vi "Set Default S Parameter Report Parameters.vi"() -> (2 "Report Variables":T1={"REPORT_TDR_PATH"="Sxx Report.TDR", "ROOT_PATH"="", "PLOT1_TDM_PATH"="", "REPORT_PDF_PATH"="", "PLOT1_RUN_ID"=1, "PLOT_STYLE"=0, "COMPANY_ID_TXT"="Summitek", "DATETIME_TXT"="", "OPERATOR_TXT"="", "SERIALNUMBER_TXT"="", "MODELNUMBER_TXT"="", "SEQID_TXT"="", "INSTRID_TXT"="", "CUSTOMTXT 1"="", "CUSTOMTXT 2"="", "CUSTOMTXT 3"="", "CUSTOMTXT 4"="", "CUSTOMTXT 5"="", "CUSTOMTXT 6"="", "CUSTOMTXT 7"="", "CUSTOMTXT 8"="", "CUSTOMTXT 9"="", "CUSTOMTXT 10"="", "PLOT1_LABEL_TXT"="", "PLOT1_Y_TXT"="", "PLOT1_X_TXT"="", "PLOT2_LABEL_TXT"="", "PLOT2_Y_TXT"="", "PLOT2_X_TXT"="", "REPORTFOOTER"="", "PLOT1_FORMAT"=0, "PLOT1_LINETYPE"=1, "PLOT1_CURVES"=[], "PLOT1_AUTO_X"=1, "PLOT1_XMIN"=0.0, "PLOT1_XMAX"=0.0, "PLOT1_X_UNIT"=2, "PLOT1_AUTO_Y"=1, "PLOT1_YMIN"=0.0, "PLOT1_YMAX"=0.0, "PLOT2_FORMAT"=0, "PLOT2_LINETYPE"=1, "PLOT2_CURVES"=[], "PLOT2_AUTO_X"=1, "PLOT2_XMIN"=0.0, "PLOT2_XMAX"=0.0, "PLOT2_X_UNIT"=2, "PLOT2_AUTO_Y"=1, "PLOT2_YMIN"=0.0, "PLOT2_YMAX"=0.0, "PRINTER"="", "CUSTOMTXT 11"="", "CUSTOMTXT 12"="", "CUSTOMTXT 13"="", "CUSTOMTXT 14"="", "CUSTOMTXT 15"="", "CUSTOMTXT 16"="", "CUSTOMTXT 17"="", "CUSTOMTXT 18"="", "CUSTOMTXT 19"="", "CUSTOMTXT 20"="", "Custom_Count"=0, "PLOT1_MARKERS"=[], "PLOT2_MARKERS"=[], "S2P"=1, "ASCII"=1} {"PLOT2_X_UNIT" items=["Hz", "kHz", "MHz", "GHz"]; "PLOT2_FORMAT" items=["Log Magnitude", "Phase", "Delay", "Linear Magnitude", "VSWR", "Insertion Loss", "Isolation", "Return Loss", "Expanded Phase"]; "PLOT1_X_UNIT" items=["Hz", "kHz", "MHz", "GHz"]; "PLOT1_FORMAT" items=["Log Magnitude", "Phase", "Delay", "Linear Magnitude", "VSWR", "Insertion Loss", "Isolation", "Return Loss", "Expanded Phase"]; "PLOT_STYLE" items=["PDF", "HTML"]})   [LabVIEW 2011]
uses:
  server/DIAdem/Datasheet/Datasheet Sxx Parameters.ctl
  server/DIAdem/Datasheet/Datasheet Sxx Plot Formats.ctl
  server/DIAdem/Datasheet/Datasheet Sxx Plot Control.ctl
  server/DIAdem/Datasheet/Datasheet Sxx Frequency Units.ctl
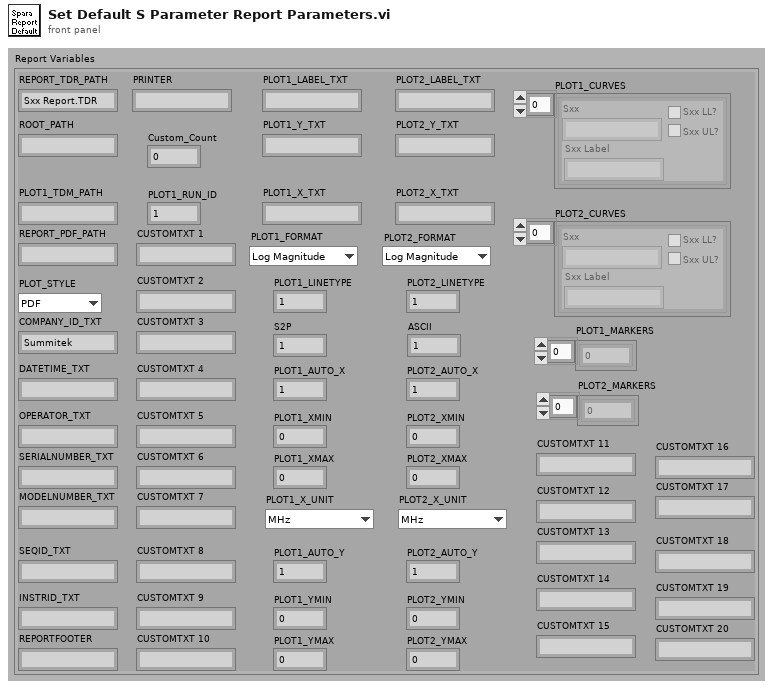
[diagram p1: front panel]
types:
  T1 = typedef "DATASHEET Sxx Parameters.ctl" = cluster{"REPORT_TDR_PATH":string, "ROOT_PATH":string, "PLOT1_TDM_PATH":string, "REPORT_PDF_PATH":string, "PLOT1_RUN_ID":i32, "PLOT_STYLE":u16, "COMPANY_ID_TXT":string, "DATETIME_TXT":string, "OPERATOR_TXT":string, "SERIALNUMBER_TXT":string, "MODELNUMBER_TXT":string, "SEQID_TXT":string, "INSTRID_TXT":string, "CUSTOMTXT 1":string, "CUSTOMTXT 2":string, "CUSTOMTXT 3":string, "CUSTOMTXT 4":string, "CUSTOMTXT 5":string, "CUSTOMTXT 6":string, "CUSTOMTXT 7":string, "CUSTOMTXT 8":string, "CUSTOMTXT 9":string, "CUSTOMTXT 10":string, "PLOT1_LABEL_TXT":string, "PLOT1_Y_TXT":string, "PLOT1_X_TXT":string, "PLOT2_LABEL_TXT":string, "PLOT2_Y_TXT":string, "PLOT2_X_TXT":string, "REPORTFOOTER":string, "PLOT1_FORMAT":T2, "PLOT1_LINETYPE":i32, "PLOT1_CURVES":T3[], "PLOT1_AUTO_X":i32, "PLOT1_XMIN":dbl, "PLOT1_XMAX":dbl, "PLOT1_X_UNIT":T4, "PLOT1_AUTO_Y":i32, "PLOT1_YMIN":dbl, "PLOT1_YMAX":dbl, "PLOT2_FORMAT":T2, "PLOT2_LINETYPE":i32, "PLOT2_CURVES":T3[], "PLOT2_AUTO_X":i32, "PLOT2_XMIN":dbl, "PLOT2_XMAX":dbl, "PLOT2_X_UNIT":T4, "PLOT2_AUTO_Y":i32, "PLOT2_YMIN":dbl, "PLOT2_YMAX":dbl, "PRINTER":string, "CUSTOMTXT 11":string, "CUSTOMTXT 12":string, "CUSTOMTXT 13":string, "CUSTOMTXT 14":string, "CUSTOMTXT 15":string, "CUSTOMTXT 16":string, "CUSTOMTXT 17":string, "CUSTOMTXT 18":string, "CUSTOMTXT 19":string, "CUSTOMTXT 20":string, "Custom_Count":i32, "PLOT1_MARKERS":dbl[], "PLOT2_MARKERS":dbl[], "S2P":i32, "ASCII":i32}
  T2 = typedef "DATASHEET Sxx Plot Formats.ctl" = u16
  T3 = typedef "DATASHEET Sxx Plot Control.ctl" = cluster{"Sxx":string, "Sxx LL?":bool, "Sxx UL?":bool, "Sxx Label":string}
  T4 = typedef "DATASHEET Sxx Frequency Units.ctl" = u16
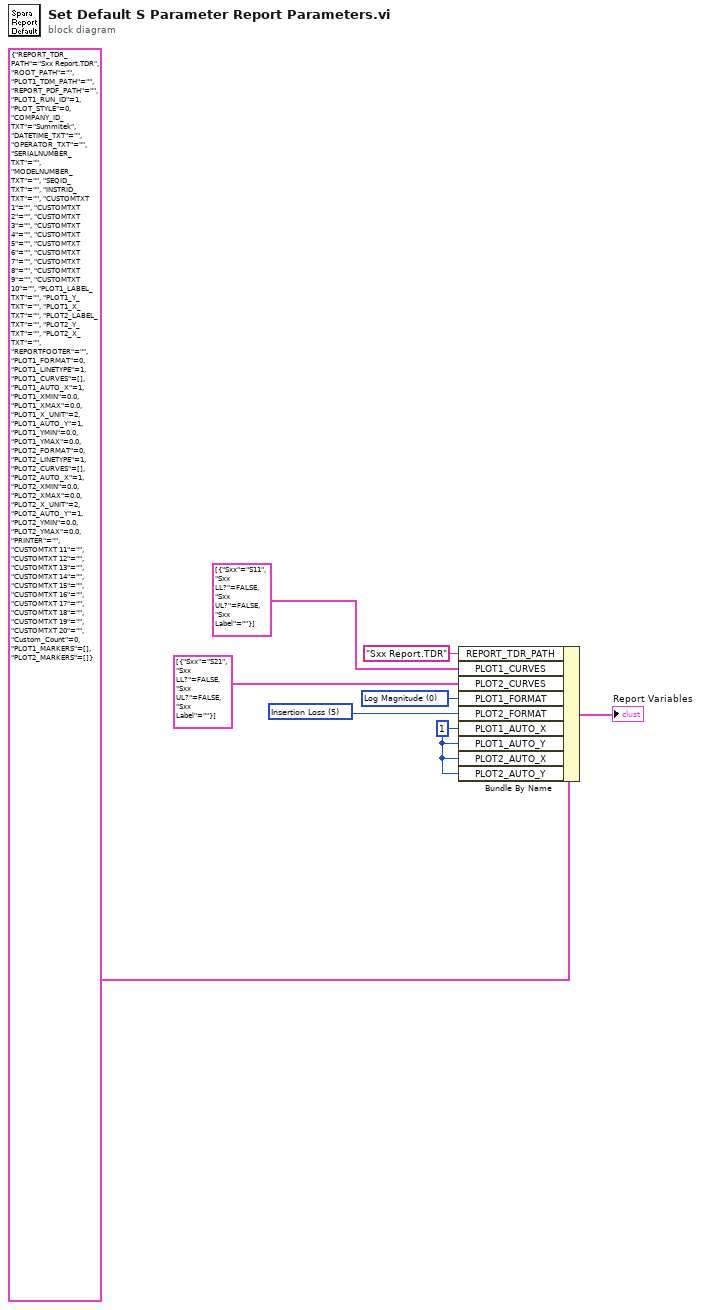
[diagram p0: block diagram]
diagram:
  w3 = 1 ("PLOT1_AUTO_X")
  w4 = T2 5 items=["Log Magnitude", "Phase", "Delay", "Linear Magnitude", "VSWR", "Insertion Loss", "Isolation", "Imaginary"] ("PLOT1_FORMAT")
  w5 = T2 0 items=["Log Magnitude", "Phase", "Delay", "Linear Magnitude", "VSWR", "Insertion Loss", "Isolation", "Imaginary"] ("PLOT1_FORMAT")
  n1 = Bundle By Name(cluster=T1 {"REPORT_TDR_PATH"="Sxx Report.TDR", "ROOT_PATH"="", "PLOT1_TDM_PATH"="", "REPORT_PDF_PATH"="", "PLOT1_RUN_ID"=1, "PLOT_STYLE"=0, "COMPANY_ID_TXT"="Summitek", "DATETIME_TXT"="", "OPERATOR_TXT"="", "SERIALNUMBER_TXT"="", "MODELNUMBER_TXT"="", "SEQID_TXT"="", "INSTRID_TXT"="", "CUSTOMTXT 1"="", "CUSTOMTXT 2"="", "CUSTOMTXT 3"="", "CUSTOMTXT 4"="", "CUSTOMTXT 5"="", "CUSTOMTXT 6"="", "CUSTOMTXT 7"="", "CUSTOMTXT 8"="", "CUSTOMTXT 9"="", "CUSTOMTXT 10"="", "PLOT1_LABEL_TXT"="", "PLOT1_Y_TXT"="", "PLOT1_X_TXT"="", "PLOT2_LABEL_TXT"="", "PLOT2_Y_TXT"="", "PLOT2_X_TXT"="", "REPORTFOOTER"="", "PLOT1_FORMAT"=0, "PLOT1_LINETYPE"=1, "PLOT1_CURVES"=[], "PLOT1_AUTO_X"=1, "PLOT1_XMIN"=0.0, "PLOT1_XMAX"=0.0, "PLOT1_X_UNIT"=2, "PLOT1_AUTO_Y"=1, "PLOT1_YMIN"=0.0, "PLOT1_YMAX"=0.0, "PLOT2_FORMAT"=0, "PLOT2_LINETYPE"=1, "PLOT2_CURVES"=[], "PLOT2_AUTO_X"=1, "PLOT2_XMIN"=0.0, "PLOT2_XMAX"=0.0, "PLOT2_X_UNIT"=2, "PLOT2_AUTO_Y"=1, "PLOT2_YMIN"=0.0, "PLOT2_YMAX"=0.0, "PRINTER"="", "CUSTOMTXT 11"="", "CUSTOMTXT 12"="", "CUSTOMTXT 13"="", "CUSTOMTXT 14"="", "CUSTOMTXT 15"="", "CUSTOMTXT 16"="", "CUSTOMTXT 17"="", "CUSTOMTXT 18"="", "CUSTOMTXT 19"="", "CUSTOMTXT 20"="", "Custom_Count"=0, "PLOT1_MARKERS"=[], "PLOT2_MARKERS"=[], "S2P"=0, "ASCII"=0} ("Report Variables"), "REPORT_TDR_PATH"="Sxx Report.TDR", "PLOT1_CURVES"=T3[] [{"Sxx"="S11", "Sxx LL?"=FALSE, "Sxx UL?"=FALSE, "Sxx Label"=""}], "PLOT2_CURVES"=T3[] [{"Sxx"="S21", "Sxx LL?"=FALSE, "Sxx UL?"=FALSE, "Sxx Label"=""}] ("PLOT1_CURVES"), "PLOT1_FORMAT"=w5, "PLOT2_FORMAT"=w4, "PLOT1_AUTO_X"=w3, "PLOT1_AUTO_Y"=w3, "PLOT2_AUTO_X"=w3, "PLOT2_AUTO_Y"=w3) -> (→"Report Variables":T1)
